vi "InsertNewData.vi"(2 "Vessel Number":i32, 3 "Time Indx":i32, 4 "New Frm #":dbl, 5 "Frm Array":dbl[][](array[numeric]), 6 "New Dpp":dbl, 7 "Dpp Array":dbl[][](array[numeric])) -> (0 "Frm Array out":dbl[][](array[numeric]), 1 "Dpp Array out":dbl[][](array[numeric]))   [LabVIEW 2019]
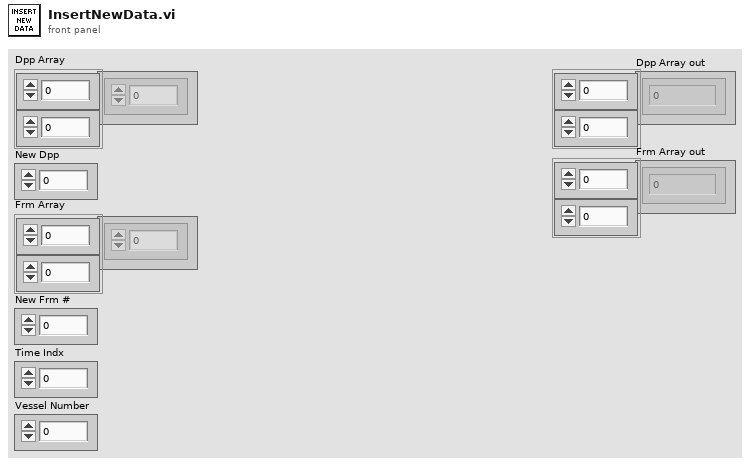
[diagram p1: front panel]
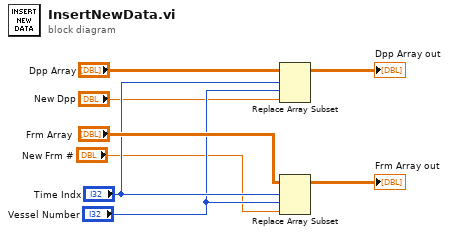
[diagram p0: block diagram]
diagram:
  n1 = Replace Array Subset(array="Dpp Array", new element="New Dpp", index (row)="Time Indx", index (col)="Vessel Number") -> (→"Dpp Array out":dbl[][])
  n2 = Replace Array Subset(array="Frm Array", new element="New Frm #", index (row)="Time Indx", index (col)="Vessel Number") -> (→"Frm Array out":dbl[][])
